vi "Build Output Folder.vi"(7 "PPT path":path, 8 "error in (no error)":errorcluster, 11 "Slide Information in":T1) -> (0 "error out":errorcluster, 2 "Output path":path, 3 "Slide Information out":T1)   [LabVIEW 2015]
uses:
  Slide Info..cluster.ctl
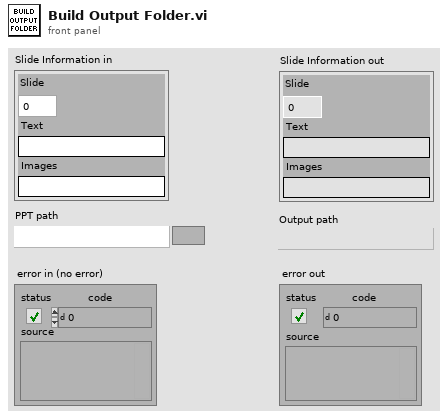
[diagram p1: front panel]
types:
  T1 = typedef "Slide Info..cluster.ctl" = cluster{"Slide":i32, "Text":string, "Images":string}
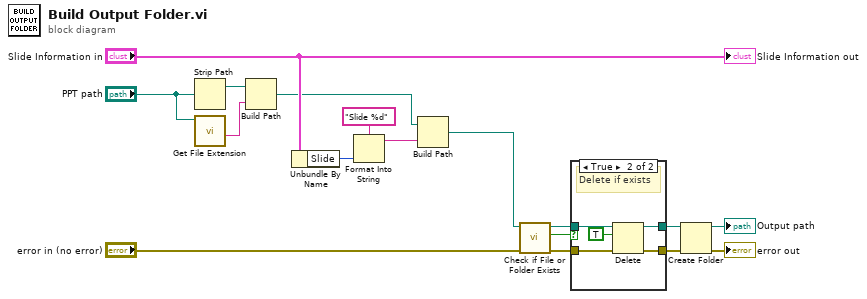
[diagram p0: block diagram]
diagram:
  n1 = Strip Path(path="PPT path") -> (stripped path=w10:path)  [unwired: 1 out]
  n2 = call <vilib>:"Get File Extension.vi"("file"="PPT path") -> ("filename without extension"=w9:string)  [unwired: 6 in, 4 out]
  n3 = Build Path(base path=w10, name or relative path=w9) -> (appended path=w8:path)
  n4 = Unbundle By Name("Slide Information in") -> ("Slide"=w15:i32)
  n5 = Format Into String(format string="Slide %d", w15) -> (resulting string=w14:string)  [unwired: 2 in, 1 out]
  n6 = Build Path(base path=w8, name or relative path=w14) -> (appended path=w1:path)
  n7 = call <vilib>:"Check if File or Folder Exists.vi"("error in (no error)"="error in (no error)", "path"=w1) -> ("error out"=w7:errorcluster, "file or folder exists?"=w6:bool, "dup path"=w5:path)  [unwired: 7 in]
  n8 = case shown="True" w6 {
    tunnel: w5 -> [w18 w24]
    tunnel: w7 -> [w19 w23]
    tunnel: [w19 w22] -> w2
    tunnel: [w18 w21] -> w4
    frame False {
    }
    frame True {
      # "Delete if exists"
      n9 = Delete(path (use dialog)=w24, entire hierarchy (F)=TRUE, error in=w23) -> (deleted path=w21:path, error out=w22:errorcluster)  [unwired: 2 in, 1 out]
    }
  }
  n10 = Create Folder(path (use dialog)=w4, error in=w2) -> (created path=→"Output path":path, error out=→"error out":errorcluster)  [unwired: 1 in, 1 out]
  "Slide Information out" <- "Slide Information in"
